vi "STM_Status_v4_development.vi"() -> ()   [LabVIEW 2014]
uses:
  <userlib>/Nanonis Prog Interface V5/Nanonis Prog Interface.lvlib
panel:
  out "LL [mBar]":dbl=1.3078783889231005e-10 format="%#.2g"
  in  "dimension size":i32=10000
  out "LL pressure":cluster{"Array out":timestamp[], "Array":dbl[]}(graph)
  out "max value STM":dbl=1.3091110140361906e-10
  out "max value prep":dbl=1.0074723173769673e-12
  in  "Emission Current":u16(ring) items=["10", "1", "0.1"]
  out "STM [mBar]":dbl=1.3078783889231005e-10 format="%#.2g"
  out "Prep [mBar]":dbl=1.0074723173769673e-12 format="%#.2g"
  out "Pressure":cluster{timestamp[], dbl[]}[](graph)
  out "Cryo [K]":dbl=4.233 format="%#.2g"
  out "STM [K]":dbl=4.658 format="%#.2g"
  out "Temperature":cluster{timestamp[], dbl[]}[](graph)
  in  "stop":bool
  in  "refresh [s]":dbl=1.0
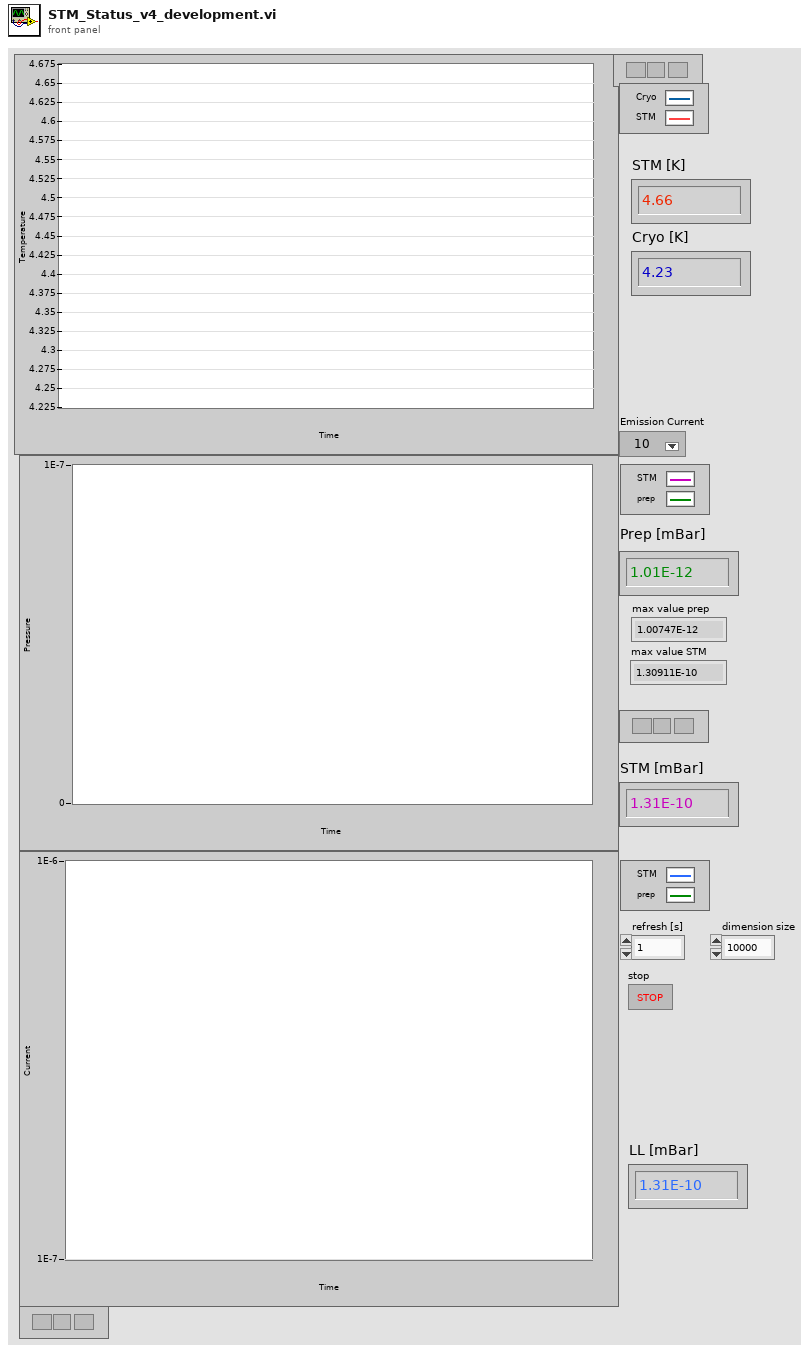
[diagram p1: front panel]
types:
  T1 = cluster{"Array out":timestamp[], "Array":dbl[]}[]
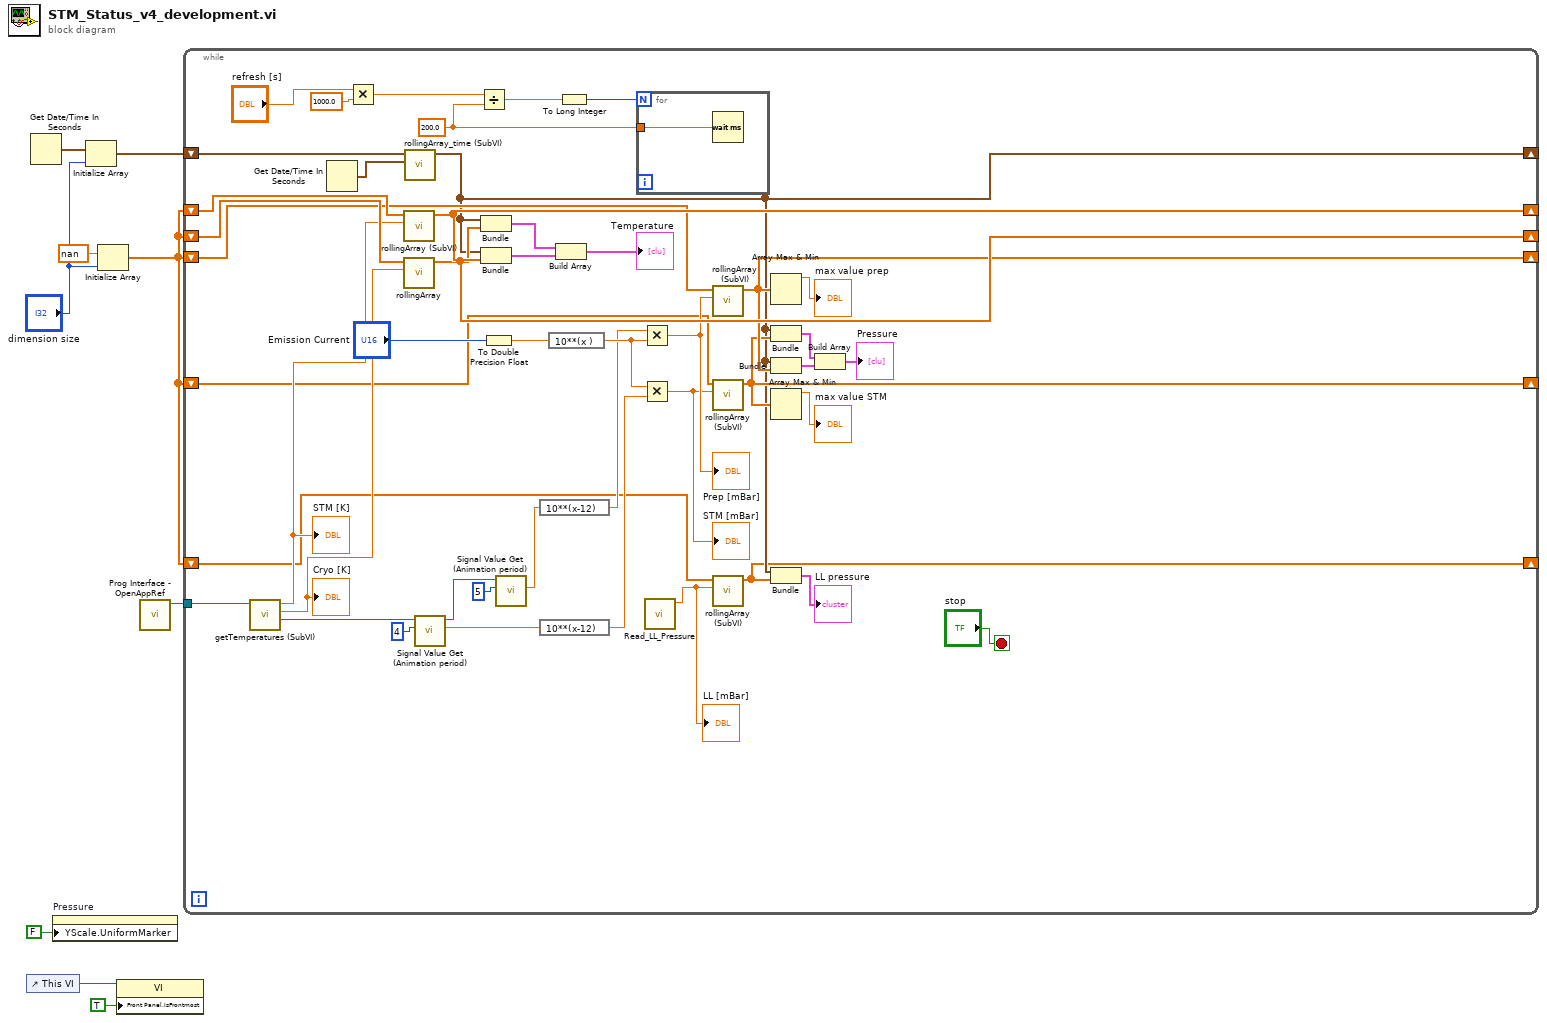
[diagram p0: block diagram]
diagram:
  n1 = control-ref of="This VI"() -> (w8:refnum<vi>)
  n2 = Get Date/Time In Seconds() -> (seconds since 1Jan1904=w3:timestamp)
  n3 = property on="Pressure" class="XYGraph (strict)"("YScale.UniformMarker"=FALSE ("Y Scale.Uniform Marker Spacing?")) -> ()  [unwired: 2 in, 2 out]
  n4 = Initialize Array(w3, "dimension size") -> (w5:timestamp[])
  n5 = Initialize Array(nan ("element"), "dimension size") -> (w2:dbl[])
  n6 = property class="VI"(reference=w8, "Front Panel.IsFrontmost"=TRUE ("Front Panel Window:Is Frontmost")) -> ()  [unwired: 1 in, 2 out]
  n7 = call <userlib>:"Prog Interface - OpenAppRef.vi"() -> ("Application reference"=w9:refnum<vi>)  [unwired: 6 in, 1 out]
  n8 = while {
    tunnel: w9 -> [w50]
    shift-right: [w17] -> _
    shift-left: w5 -> [w53]
    shift-right: [w55] -> _
    shift-left: w2 -> [w52]
    shift-right: [w54] -> _
    shift-left: w2 -> [w51]
    shift-right: [w20] -> _
    shift-left: w2 -> [w21]
    shift-right: [w49] -> _
    shift-left: w2 -> [w48]
    shift-right: [w15] -> _
    shift-left: w2 -> [w18]
    stop <- "stop" stop-if-true
    w12 = 200.0 ("y")
    n9 = call "getTemperatures (SubVI).vi"("Application in"=w50) -> ("Application ref out"=w33:refnum<vi>, "TCryo"=w24:dbl, "TSTM"=w27:dbl)  [unwired: 7 in, 1 out]
    "STM [K]" <- w27
    "Cryo [K]" <- w24
    n10 = Get Date/Time In Seconds() -> (seconds since 1Jan1904=w25:timestamp)
    n11 = Multiply(x="refresh [s]", y=1000.0) -> (x*y=w14:dbl)
    n12 = call "rollingArray (SubVI).vi"("new element/subarray"=w27, "array"=w52) -> ("Array"=w55:dbl[])  [unwired: 9 in]
    n13 = call-poly "rollingArray.vi"("new element/subarray"=w24, "array"=w51) -> ("Array"=w54:dbl[])  [unwired: 9 in]
    n14 = call "rollingArray_time (SubVI).vi"("seconds since 1Jan1904"=w25, "Array in"=w53) -> ("Array out"=w17:timestamp[])  [unwired: 9 in]
    n15 = call <userlib>:"Signal Value Get (Animation period).vi"("Signal index (0-47)"=i8 4, "Application ref in"=w33) -> ("Signal value"=w34:sgl, "Application ref out"=w40:refnum<vi>)  [unwired: 6 in, 1 out]
    n16 = Divide(x=w14, y=w12) -> (x/y=w13:dbl)
    n17 = Bundle("Array out"=w17, "Array"=w54) -> (w43:cluster{"Array out":timestamp[], "Array":dbl[]})  [unwired: 1 in]
    n18 = Bundle("Array out"=w17, "Array"=w55) -> (w42:cluster{"Array out":timestamp[], "Array":dbl[]})  [unwired: 1 in]
    n19 = To Double Precision Float(number="Emission Current") -> (double precision float=w44:dbl)
    n20 = call <userlib>:"Signal Value Get (Animation period).vi"("Signal index (0-47)"=i8 5, "Application ref in"=w40) -> ("Signal value"=w32:sgl)  [unwired: 6 in, 2 out]
    n21 = expression code="10**(x-12)"(w32) -> (w31:sgl)
    n22 = expression code="10**(x-12)"(w34) -> (w30:sgl)
    n23 = expression code="10**(x )"(w44) -> (w45:dbl)
    n24 = Build Array(w43, w42) -> (→"Temperature":T1)
    n25 = To Long Integer(number=w13) -> (32bit integer=w11:i32)
    n26 = for {
      N: w11 -> [_]
      tunnel: w12 -> [w56]
      n27 = Wait (ms)(milliseconds to wait=w56) -> ()  [unwired: 1 out]
    }
    n28 = Multiply(x=w31, y=w45) -> (x*y=w26:dbl)
    "Prep [mBar]" <- w26
    n29 = Multiply(x=w45, y=w30) -> (x*y=w19:dbl)
    "STM [mBar]" <- w19
    n30 = call "Read_LL_Pressure.vi"() -> ("LL Pressure"=w10:dbl)  [unwired: 11 in]
    "LL [mBar]" <- w10
    n31 = call "rollingArray (SubVI).vi"("new element/subarray"=w26, "array"=w48) -> ("Array"=w49:dbl[])  [unwired: 9 in]
    n32 = call "rollingArray (SubVI).vi"("new element/subarray"=w19, "array"=w21) -> ("Array"=w20:dbl[])  [unwired: 9 in]
    n33 = call "rollingArray (SubVI).vi"("new element/subarray"=w10, "array"=w18) -> ("Array"=w15:dbl[])  [unwired: 9 in]
    n34 = Array Max & Min(array=w49) -> (max value=→"max value prep":dbl)  [unwired: 3 out]
    n35 = Bundle("Array out"=w17, "Array"=w20) -> (w37:cluster{"Array out":timestamp[], "Array":dbl[]})  [unwired: 1 in]
    n36 = Bundle("Array out"=w17, "Array"=w49) -> (w36:cluster{"Array out":timestamp[], "Array":dbl[]})  [unwired: 1 in]
    n37 = Array Max & Min(array=w20) -> (max value=→"max value STM":dbl)  [unwired: 3 out]
    n38 = Bundle("Array out"=w17, "Array"=w15) -> (→"LL pressure":cluster{"Array out":timestamp[], "Array":dbl[]})  [unwired: 1 in]
    n39 = Build Array(w37, w36) -> (→"Pressure":T1)
  }
